vi "MainDeQueue.vi"(6 "timeout in ms (-1)":i32=-1, 8 "error in":errorcluster) -> (0 "error out":errorcluster, 1 "timed out?":bool, 3 "States":T1)   [LabVIEW 2022 SP3]
uses:
  Type Def/MainStates Cluster.ctl
  Type Def/MainStates.ctl
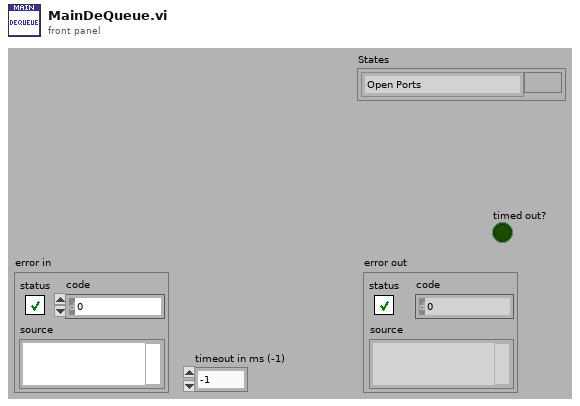
[diagram p1: front panel]
types:
  T1 = typedef "MainStates Cluster.ctl" = cluster{"States":T2, "Data":variant}
  T2 = typedef "MainStates.ctl" = enum16{"Open Ports", "Close Ports", "Main", "Settings", "Voltaje", "Probe", "Lenguaje", "Callibration", "Exit", "Voltage Test", "Test 2", "End test"}
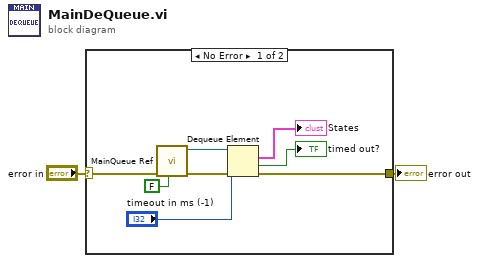
[diagram p0: block diagram]
diagram:
  n1 = case shown="No Error" "error in" {
    selector: "error in" -> [w9 w11]
    tunnel: [w7 w11] -> w1
    frame No Error {
      n2 = call "MainQueue Ref.vi"("Write:T/Read:(F)"=FALSE ("Write:T/Read:F"), "error in"=w9) -> ("error out"=w8:errorcluster, "queue out"=w6:refnum<queue>)  [unwired: 8 in]
      n3 = Dequeue Element(queue=w6, timeout in ms (-1)="timeout in ms (-1)", error in (no error)=w8) -> (element=→"States":T1, timed out?=→"timed out?":bool, error out=w7:errorcluster)  [unwired: 1 out]
    }
    frame Error {
    }
  }
  "error out" <- w1
